vi "Operation UI.vi"(0 "Subtract in":refnum<class "Subtract.lvclass">, 5 "A":dbl, 7 "B":dbl, 9 "Calculate":bool, 11 "Error In":errorcluster, 12 "Stop":refnum<user-event>, 13 "Class Data":refnum<user-event>) -> (4 "Subtract out":refnum<class "Subtract.lvclass">, 6 "C":dbl, 15 "Error Out":errorcluster)   [LabVIEW 2023, in "Subtract.lvclass"]
doc: "The VI contains the addition operation UI that accepts two input numbers and performs subtraction operation and displays the output when user clicks calculate button"
uses:
  Subtract.lvclass
  C:/Users/Ancy.Augustin/Downloads/LVOOPS DVR/LVOOPS DVR/Classes/Arithemtic Operation/Arithemetic Operation.lvclass
  Arithemtic Operation/Arithemetic Operation.lvclass
  Typedef/User Event Operations.ctl
panel:
  # "SUBTRACTION"
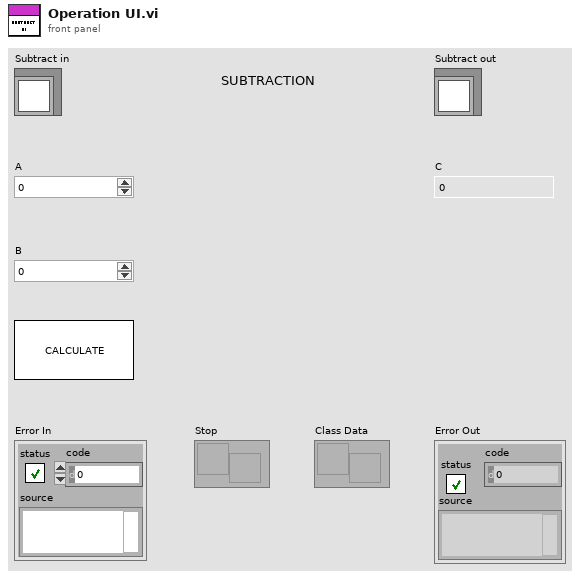
[diagram p1: front panel]
types:
  T1 = typedef "User Event Operations.ctl" = enum16{"Obtain", "Generate", "Release"}
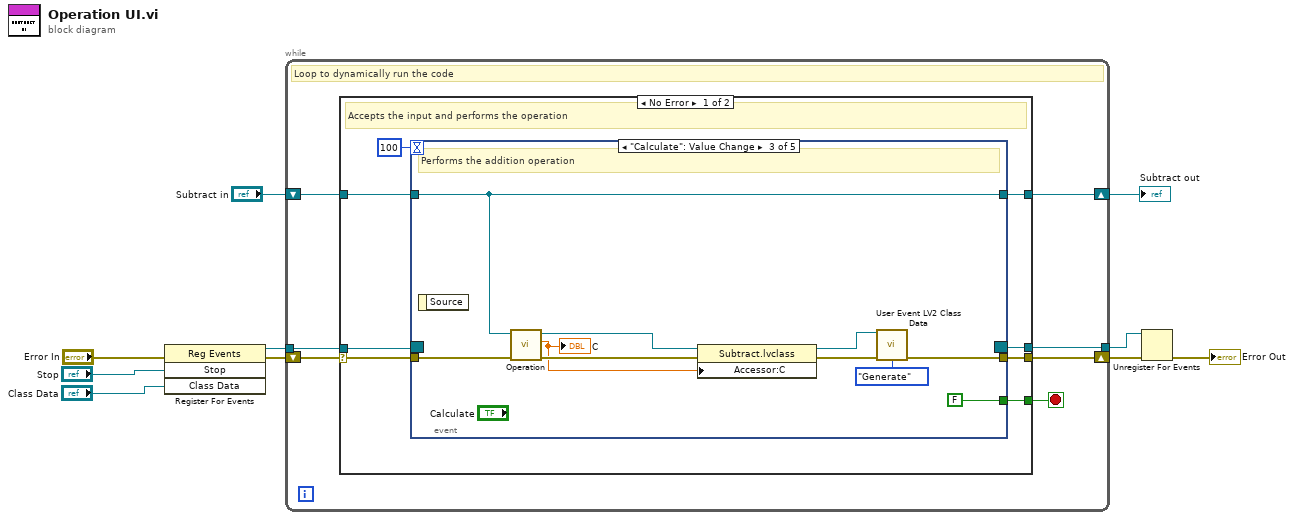
[diagram p0: block diagram]
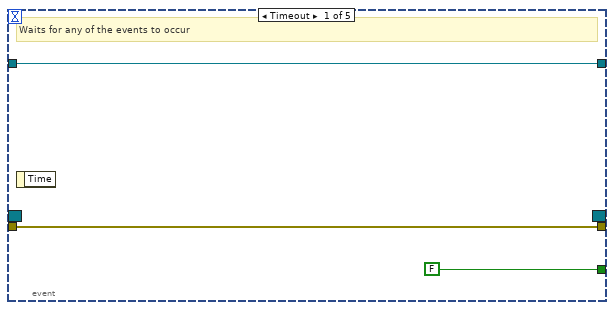
[diagram p2: hidden frame]
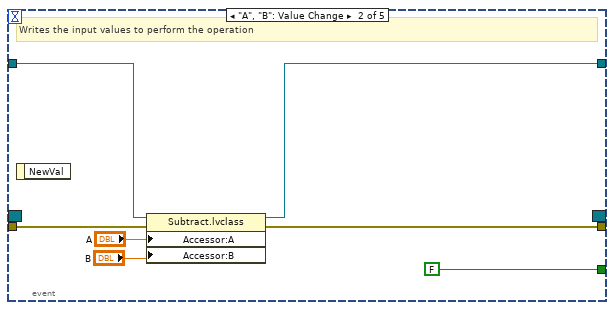
[diagram p3: hidden frame]
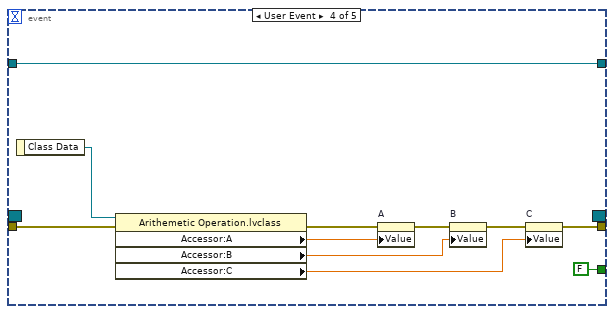
[diagram p4: hidden frame]
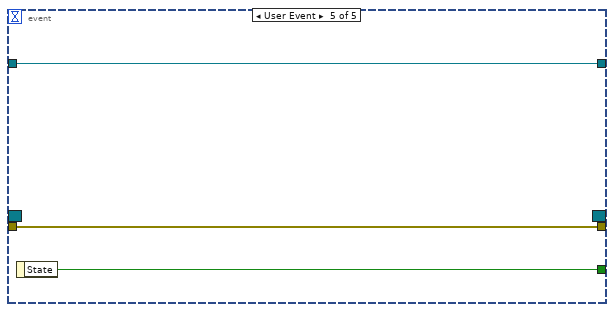
[diagram p5: hidden frame]
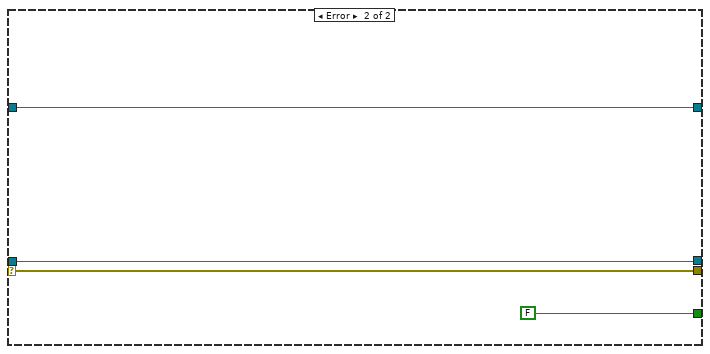
[diagram p6: hidden frame]
diagram:
  n1 = register-events(error in="Error In", "Stop", "Class Data") -> (reference out=w7:refnum<event-registration>, error out=w8:errorcluster)  [unwired: 1 in]
  n2 = while {
    shift-right: [w16] -> w10
    shift-left: w8 -> [w17]
    shift-right: [w14] -> w3
    shift-left: "Subtract in" -> [w15]
    tunnel: w7 -> [w13]
    tunnel: [w12] -> w5
    stop <- w11 stop-if-true
    # "Loop to dynamically run the code"
    n3 = case shown="No Error" w17 {
      selector: w17 -> [w23 w63]
      tunnel: [w22 w63] -> w16
      tunnel: [w24 w62] -> w14
      tunnel: w15 -> [w25 w62]
      tunnel: w13 -> [w20 w61]
      tunnel: [w19 w61] -> w12
      tunnel: [w18 FALSE] -> w11
      frame No Error {
        # "Accepts the input and performs the operation"
        n4 = event shown="[2] \"Calculate\": Value Change" {
          selector: w20 -> [_ _ _ _ _]
          dyn-events: [_ _ _ _ _] -> w19
          timeout: 100 -> [_ _ _ _ _]
          tunnel: [w28 w30 w38 w56 w59] -> w24
          tunnel: w25 -> [w28 w33 w38 w56 w59]
          tunnel: w23 -> [w27 w35 w45 w55 w58]
          tunnel: [w27 w34 w42 w50 w58] -> w22
          tunnel: [FALSE FALSE FALSE FALSE w57] -> w18
          event Timeout {
            # "Waits for any of the events to occur"
            n5 = event-data() -> ()  [unwired: 1 in, 1 out]
          }
          event "A", "B": Value Change {
            # "Writes the input values to perform the operation"
            n6 = event-data() -> ()  [unwired: 1 in, 1 out]
            n7 = property class="Subtract.lvclass"(reference=w33, error in=w35, "Accessor:A"="A", "Accessor:B"="B") -> (reference out=w30:refnum<class "Subtract.lvclass">, error out=w34:errorcluster)
          }
          event "Calculate": Value Change {
            # "Performs the addition operation"
            n8 = event-data() -> ()  [unwired: 1 in, 1 out]
            n9 = call-dynamic "Operation.vi"("Error In"=w45, "Subtract in"=w38) -> ("Error Out"=w44:errorcluster, "C"=w39:dbl, "Subtract out"=w40:refnum<class "Subtract.lvclass">)  [unwired: 7 in]
            "C" <- w39
            n10 = property class="Subtract.lvclass"(reference=w40, error in=w44, "Accessor:C"=w39) -> (reference out=w37:refnum<class "Subtract.lvclass">, error out=w41:errorcluster)
            n11 = call "User Event LV2 Class Data.vi"("Class Data"=w37, "Error In"=w41, "Operation"=User_Event_Operations."Generate") -> ("Error Out"=w42:errorcluster)  [unwired: 11 in, 1 out]
          }
          event User Event {
            n12 = event-data() -> ("Class Data"=w52:refnum<class "Arithemetic Operation.lvclass">)  [unwired: 1 in]
            n13 = property class="Arithemetic Operation.lvclass"(reference=w52, error in=w55) -> (error out=w54:errorcluster, "Accessor:A"=w49:dbl, "Accessor:B"=w48:dbl, "Accessor:C"=w47:dbl)  [unwired: 1 out]
            n14 = property on="A" class="DigNum (strict)"(error in=w54, "Value"=w49) -> (error out=w53:errorcluster)  [unwired: 1 in, 1 out]
            n15 = property on="B" class="DigNum (strict)"(error in=w53, "Value"=w48) -> (error out=w51:errorcluster)  [unwired: 1 in, 1 out]
            n16 = property on="C" class="DigNum (strict)"(error in=w51, "Value"=w47) -> (error out=w50:errorcluster)  [unwired: 1 in, 1 out]
          }
          event User Event {
            n17 = event-data() -> ("State"=w57:bool)  [unwired: 1 in]
          }
        }
      }
      frame Error {
      }
    }
  }
  "Subtract out" <- w3
  n18 = Unregister For Events(event registration refnum=w5, error in=w10) -> (error out=→"Error Out":errorcluster)
